vi "stage_initialise_PI_Mecury.vi"(9 "Referenz Modus":bool, 10 "Referenzierung erzwingen":bool, 11 "SN von Controller 1":string="0135500571") -> (0 "error out":errorcluster, 2 "Aktuelle xyz-Position":dbl[](array[numeric]) format="%#.6g", 3 "Bühnen initialisiert":bool)   [LabVIEW 2009]
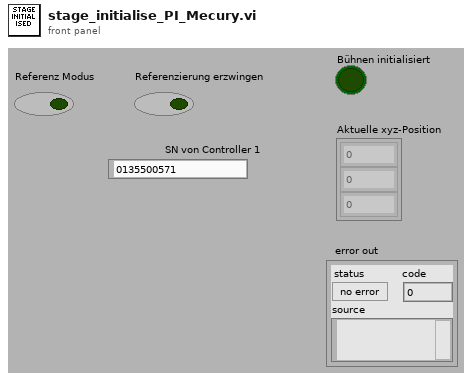
[diagram p1: front panel]
types:
  T1 = cluster{"Register DC":bool, "DaisyChain Search?":bool, "Device ID":i32}
  T2 = cluster{"SN von Controller 1":string, "USB Search?":bool}
  T3 = cluster{"RON Affected axes":string[], bool[], bool}
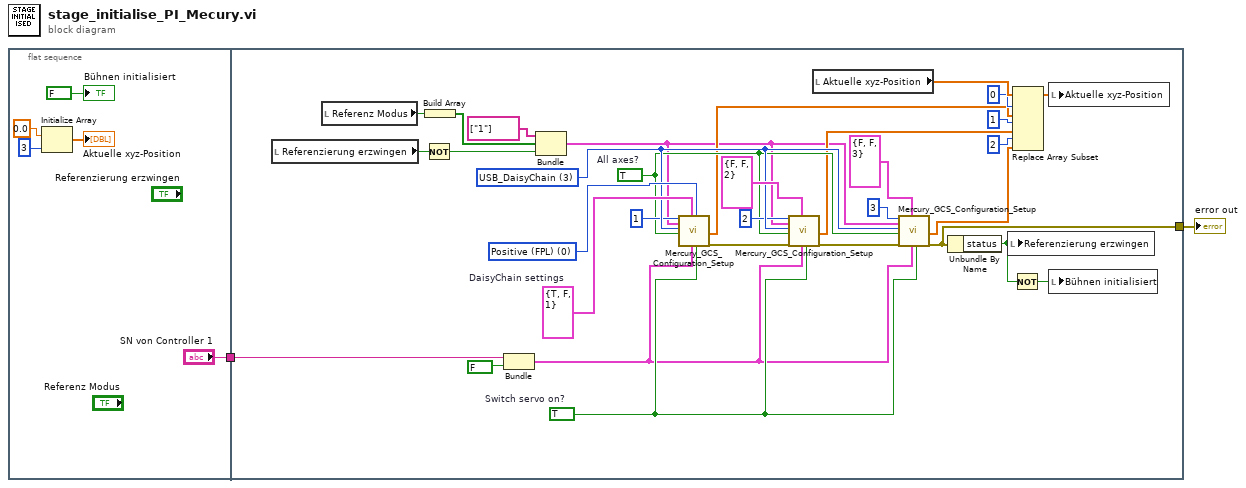
[diagram p0: block diagram]
diagram:
  n1 = flat-sequence {
    tunnel: ["SN von Controller 1"] -> w2
    tunnel: [w24] -> w1
    tunnel: w2 -> [w13]
    frame #0 {
      n2 = Initialize Array(0.0 ("Element"), 3 ("Dimension")) -> (→"Aktuelle xyz-Position":dbl[])
      "Bühnen initialisiert" <- FALSE ("NICHT x?")
    }
    frame #1 {
      w34 = TRUE  # Switch servo on?
      w38 = u16 0 items=["Positive (FPL)", "Negative (FNL)"] ("Limit switch selection")
      w28 = TRUE  # All axes?
      w35 = u16 3 items=["RS232", "RS232 DaisyChain", "USB", "USB_DaisyChain"] ("Interface")
      w39 = T1 {"Register DC"=TRUE, "DaisyChain Search?"=FALSE, "Device ID"=1}  # DaisyChain settings
      n3 = local read "Referenzierung erzwingen"() -> (w23:bool)
      n4 = local read "Referenz Modus"() -> (w10:bool)
      n5 = Not(x=w23) -> (.not. x?=w32:bool)
      n6 = Build Array(w10) -> (w9:bool[])
      n7 = Bundle("SN von Controller 1"=w13, "USB Search?"=FALSE) -> (w11:T2)  [unwired: 1 in]
      n8 = Bundle("RON Affected axes"=string[] ["1"], w9, w32) -> (w8:T3)  [unwired: 1 in]
      n9 = call "Mercury_GCS_Configuration_Setup.vi"("System no."=1, "RON settings"=w8, "Interface"=w35, "All axes?"=w28, "DaisyChain settings"=w39, "USB settings"=w11, "Reference Move"=w38, "Switch servo on?"=w34) -> ("Position"=w19:dbl[], "error out"=w26:errorcluster)  [unwired: 5 in, 5 out]
      n10 = call "Mercury_GCS_Configuration_Setup.vi"("System no."=2, "RON settings"=w8, "Interface"=w35, "All axes?"=w28, "error in"=w26, "DaisyChain settings"=T1 {"Register DC"=FALSE, "DaisyChain Search?"=FALSE, "Device ID"=2}, "USB settings"=w11, "Switch servo on?"=w34) -> ("Position"=w15:dbl[], "error out"=w25:errorcluster)  [unwired: 5 in, 5 out]
      n11 = local read "Aktuelle xyz-Position"() -> (w21:dbl[])
      n12 = call "Mercury_GCS_Configuration_Setup.vi"("System no."=3, "RON settings"=w8, "Interface"=w35, "All axes?"=w28, "error in"=w25, "DaisyChain settings"=T1 {"Register DC"=FALSE, "DaisyChain Search?"=FALSE, "Device ID"=3}, "USB settings"=w11, "Switch servo on?"=w34) -> ("Position"=w14:dbl[], "error out"=w24:errorcluster)  [unwired: 5 in, 5 out]
      n13 = Unbundle By Name(w24) -> ("status"=w22:bool)
      n14 = local write "Referenzierung erzwingen"(w22) -> ()
      n15 = Not(x=w22) -> (.not. x?=w27:bool)
      n16 = Replace Array Subset(array=w21, new element #1=w19, index #1=0 ("Index"), new element #2=w15, index #2=1 ("Index"), new element #3=w14, index #3=2 ("Index")) -> (w18:dbl[])
      n17 = local write "Aktuelle xyz-Position"(w18) -> ()
      n18 = local write "Bühnen initialisiert"(w27) -> ()
    }
  }
  "error out" <- w1
